vi "Test AMS Climate Chamber Template.vi"() -> (3 "gRPC Listening Port":i32)   [LabVIEW 2026]
uses:
  Plugin/AMS Climate Chamber Template/AMS Climate Chamber Template.lvclass
  C:/Program Files/National Instruments/LabVIEW 2026/vi.lib/ADAS Replay HIL/Template Node/Plugin/Template Node/Template Node.lvclass
  C:/Program Files/National Instruments/LabVIEW 2026/Targets/NI/RT/Linux/PXI/vi.lib/ADAS Replay HIL/AdasNode/AdasNode.lvlibp/IAdasNode/IAdasNode.lvclass
  D:/git/ams-climate-chamber-plugin-template/src/Plugin/AMS Climate Chamber Template/AMS Climate Chamber Template.lvclass
  <vilib>/ADAS Replay HIL/Template Node/Plugin/Template Node/Template Node.lvclass
  <vilib>/ADAS Replay HIL/ADAS Plugin Utilities/AdasLvTemplateSystemLog/AdasLvTemplateSystemLog.lvlib
  <vilib>/ADAS Replay HIL/Template Node/Plugin/Template Node/Common Configuration Params.ctl
  Plugin/AMS Climate Chamber Template/Configuration Params.ctl
panel:
  in  "Version":string="1.0"
  in  "Default Parameters":T1={"Common"={"Iteration Interval (s)"=0.001, "T0 (ns)"=0, "Priority"=100, "Processor"=-2, "Wait in Ready State"=TRUE}, "Amount of Channels"=0, "Address"=""} {"Common"."Iteration Interval (s)" format="%#_13g"}
  out "# of errors":i32
  in  "stop":bool
  out "Errors":errorcluster[](array[cluster])
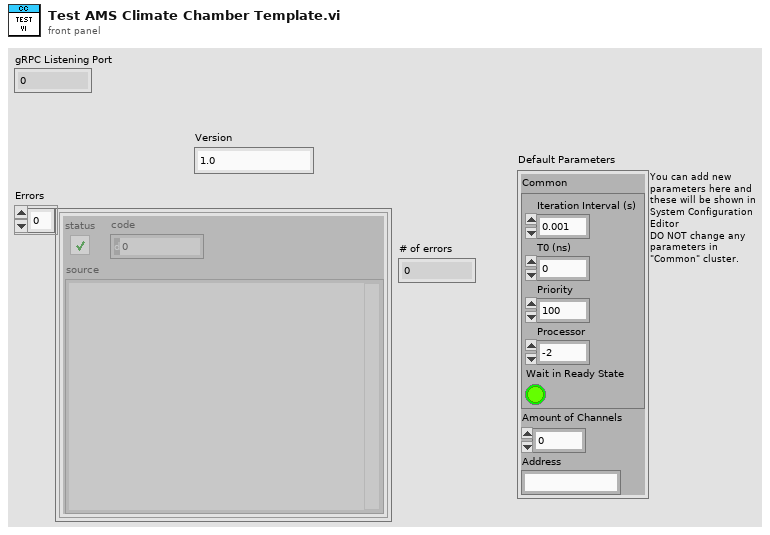
[diagram p1: front panel]
types:
  T1 = typedef "AMS Climate Chamber Template.lvlib/AMS Climate Chamber Template.lvclass/Configuration Params.ctl" = cluster{"Common":T2, "Amount of Channels":u32, "Address":string}
  T2 = typedef "Template Node.lvlib/Template Node.lvclass/Common Configuration Params.ctl" = cluster{"Iteration Interval (s)":dbl, "T0 (ns)":u64, "Priority":i32, "Processor":i32, "Wait in Ready State":bool}
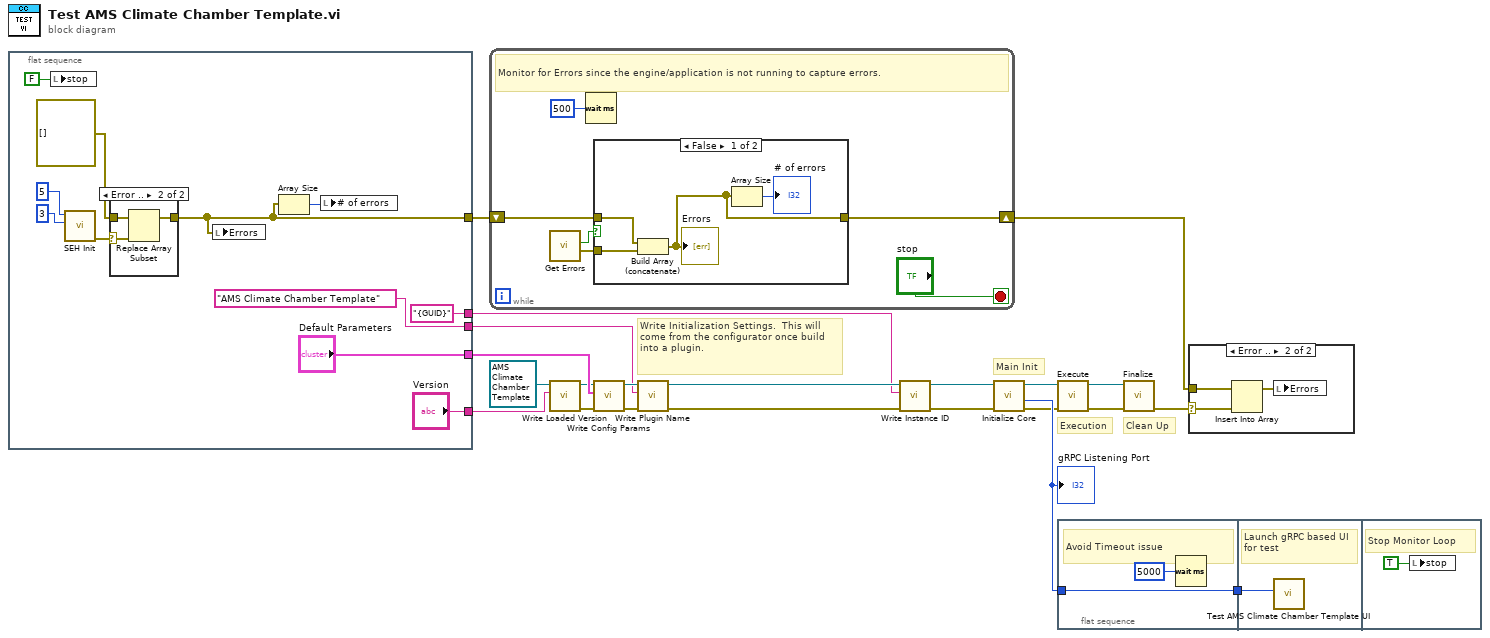
[diagram p0: block diagram]
diagram:
  # "Clean Up"
  # "Execution"
  # "Main Init"
  # "Write Initialization Settings.  This will come from the configurator once build into a plugin."
  n1 = flat-sequence {
    tunnel: ["AMS Climate Chamber Template" ("Plugin Name")] -> w16
    tunnel: ["{GUID}" ("Instance ID")] -> w15
    tunnel: ["Default Parameters"] -> w11
    tunnel: [w25] -> w8
    tunnel: ["Version"] -> w1
    frame #0 {
      n2 = local write "stop"(FALSE ("stop")) -> ()
      n3 = call <userlib>:"SEH Init.vi"("Number of Priorities"=3, "Notifications per Priority"=5) -> ("error out"=w26:errorcluster)  [unwired: 9 in]
      n4 = case shown="Error .." w26 {
        selector: w26 -> [_ w36]
        tunnel: errorcluster[] [] -> [w34 w37]
        tunnel: [w34 w35] -> w25
        frame No Error {
        }
        frame Error {
          n5 = Replace Array Subset(array=w37, new element=w36) -> (w35:errorcluster[])  [unwired: 1 in]
        }
      }
      n6 = local write "Errors"(w25) -> ()
      n7 = Array Size(array=w25) -> (size(s)=w24:i32)
      n8 = local write "# of errors"(w24) -> ()
    }
  }
  n9 = while {
    shift-right: [w40] -> w7
    shift-left: w8 -> [w43]
    stop <- "stop" stop-if-true
    # "Monitor for Errors since the engine/application is not running to capture errors."
    n10 = call <vilib>:"Get Errors.vi"() -> ("Transmitted Errors"=w38:errorcluster[], "Empty?"=w39:bool)  [unwired: 9 in, 1 out]
    n11 = Wait (ms)(milliseconds to wait=u32 500) -> ()  [unwired: 1 out]
    n12 = case shown="False" w39 {
      tunnel: w43 -> [w47 w48]
      tunnel: [w44 w48] -> w40
      tunnel: w38 -> [w46 _]
      frame False {
        n13 = Build Array (concatenate)(w47, w46) -> (w44:errorcluster[])
        "Errors" <- w44
        n14 = Array Size(array=w44) -> (size(s)=→"# of errors":i32)
      }
      frame True {
      }
    }
  }
  n15 = call <vilib>:"Write Loaded Version.vi"("Loaded Version"=w1, "Template Node in"=refnum<class "AMS Climate Chamber Template.lvclass"> refnum ("Test Node.lvlib:Test Node.lvclass")) -> ("error out"=w2:errorcluster, "Template Node out"=w3:refnum<class "AMS Climate Chamber Template.lvclass">)  [unwired: 8 in]
  n16 = call "Write Config Params.vi"("error in"=w2, "Default Parameters"=w11, "Node in"=w3) -> ("error out"=w22:errorcluster, "Node out"=w20:refnum<class "AMS Climate Chamber Template.lvclass">)  [unwired: 7 in]
  n17 = call <vilib>:"Write Plugin Name.vi"("error in"=w22, "Plugin Name"=w16, "Template Node in"=w20) -> ("error out"=w21:errorcluster, "Template Node out"=w18:refnum<class "AMS Climate Chamber Template.lvclass">)  [unwired: 7 in]
  n18 = call <vilib>:"Write Instance ID.vi"("error in"=w21, "Instance ID"=w15, "Template Node in"=w18) -> ("error out"=w19:errorcluster, "Template Node out"=w17:refnum<class "AMS Climate Chamber Template.lvclass">)  [unwired: 7 in]
  n19 = call <vilib>:"Initialize Core.vi"("error in"=w19, "Node in"=w17) -> ("error out"=w5:errorcluster, "gRPC Listening Port"=w10:i32, "Node out"=w9:refnum<class "AMS Climate Chamber Template.lvclass">)  [unwired: 7 in]
  "gRPC Listening Port" <- w10
  n20 = call-dynamic "Execute.vi"("error in (no error)"=w5, "Node in"=w9) -> ("error out"=w13:errorcluster, "Node out"=w14:refnum<class "AMS Climate Chamber Template.lvclass">)  [unwired: 6 in, 2 out]
  n21 = flat-sequence {
    tunnel: w10 -> [w50]
    tunnel: [w50] -> w4
    tunnel: w4 -> [w51]
    frame #0 {
      # "Avoid Timeout issue"
      n22 = Wait (ms)(milliseconds to wait=u32 5000) -> ()  [unwired: 1 out]
    }
    frame #1 {
      # "Launch gRPC based UI for test"
      n23 = call "Test AMS Climate Chamber Template UI.vi"("gRPC Port"=w51) -> ()  [unwired: 11 in]
    }
    frame #2 {
      # "Stop Monitor Loop"
      n24 = local write "stop"(TRUE ("stop")) -> ()
    }
  }
  n25 = call-dynamic "Finalize.vi"("error in (no error)"=w13, "Node in"=w14) -> ("error out"=w6:errorcluster)  [unwired: 9 in]
  n26 = case shown="Error .." w6 {
    selector: w6 -> [_ w54]
    tunnel: w7 -> [_ w55]
    frame No Error {
    }
    frame Error {
      n27 = Insert Into Array(array=w55, new element=w54) -> (w53:errorcluster[])  [unwired: 1 in]
      n28 = local write "Errors"(w53) -> ()
    }
  }
